vi "DLUInputBuffer.vi"(6 "Ready for Output":bool, 9 "Input Valid":bool, 10 "Input Data":T1) -> (1 "Output Data":bool, 2 "Output Data":T1, 4 "Ready For Input":bool)   [LabVIEW 2014, in "IO Node Logic Template.lvlib"]
uses:
  IO Node Logic Template.lvlib
  Node/Controls/Node_Command_Sent.ctl
  <vilib>/rvi/Emulation/niFpgaSctlEmulationGetInTimedLoop.vi
  <vilib>/rvi/DataTransferAndStorage/Container/Common/niFpgaContainerGetUniqueNameForEmu.vi
  <vilib>/rvi/DataTransferAndStorage/Container/Common/niFpgaContainerSetEmuInfo.vi
  <vilib>/rvi/eio/common/nirviEmuReportErrorAndStop.vi
  <vilib>/rvi/DataTransferAndStorage/Container/Common/niFpgaContainerExecOnDevCompGetState.vi
  <vilib>/rvi/Emulation/niFpgaEmulationIsFPGAContextNoSignature.vi
  <vilib>/rvi/errors/niFpgaSetErrorForExecOnDevCompSimple.vi
  <vilib>/rvi/FIFO/Fifo_Resource/nirvififoEmulationSetSize.vi
  <vilib>/rvi/FIFO/Fifo_Resource/nirviFifoEmulationQueueMgr.vi
  <instcachedir>/0/nirviFifoEmulationQueueMgr_E5CAEC123FF24DC58D834DCA3CDAA9B5.lvgen/nirviFifoEmulationQueueMgr_E5CAEC123FF24DC58D834DCA3CDAA9B5_001.vi
  <vilib>/rvi/FIFO/Fifo_Resource/nirvififoEmulationDetermineInputValidOut.vi
  <vilib>/rvi/FIFO/Fifo_Resource/nirvififoEmulationCreateLock.vi
  <vilib>/rvi/Emulation/niFpgaProcessEmulError.vi
  <vilib>/rvi/FIFO/Fifo_Resource/nirvififoEmulationObtainLock.vi
  <vilib>/rvi/FIFO/Fifo_Resource/nirvififoEmulationReleaseLock.vi
  <vilib>/rvi/occurrence/nirviWaitOnOccurrenceBase.vi
  <vilib>/rvi/errors/nirviReportUnexpectedCaseInternalError.vi
  <vilib>/rvi/errors/nirviReportUnexpectedCaseInternalError (U32).vi
  <vilib>/rvi/interface/RandomDataEmulation/niFpgaRandomDataHandleErrors.vi
  <vilib>/rvi/LocalResourceManager/LocalResourceManager.xnode
  <vilib>/rvi/DataTransferAndStorage/Container/XNode/niFpgaContainer.xnode
  <vilib>/rvi/FIFO/Fifo_Resource/niFpgaFifoEmulationRefIn.vi
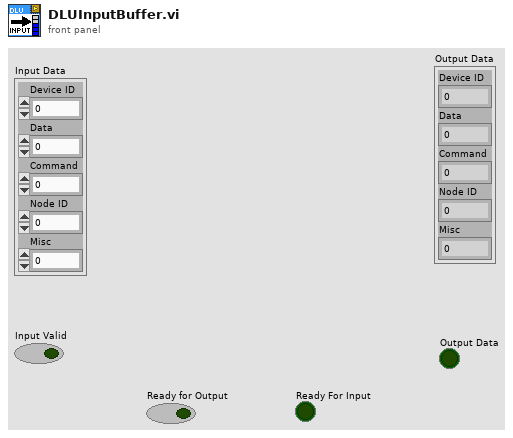
[diagram p1: front panel]
types:
  T1 = typedef "IO Node Logic Template.lvlib/Node_Command_Sent.ctl" = cluster{"Device ID":u8, "Data":u64, "Command":u8, "Node ID":u8, "Misc":u8}
  T2 = cluster{"Channel ID":u8, "Data":u64, "Command":u8, "Sender Address":u8, "Misc":u8}
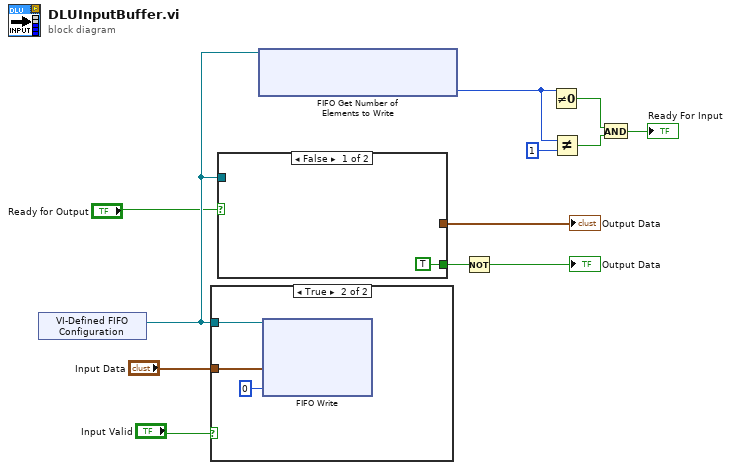
[diagram p0: block diagram]
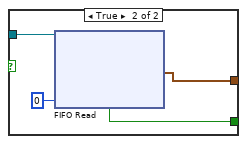
[diagram p2: hidden frame]
diagram:
  n1 = xnode "VI-Defined FIFO Configuration"() -> ("FIFO Out"=w8:refnum<k21>)
  n2 = case shown="True" "Input Valid" {
    tunnel: "Input Data" -> [_ w15]
    tunnel: w8 -> [_ w13]
    frame False {
    }
    frame True {
      n3 = xnode "FIFO Write"("Element"=w15, "Timeout"=0, "FIFO In"=w13) -> ()  [unwired: 2 out]
    }
  }
  n4 = case shown="False" "Ready for Output" {
    tunnel: [_ w19] -> w11
    tunnel: [TRUE ("Timed Out?") w18] -> w10
    tunnel: w8 -> [_ w17]
    frame False {
    }
    frame True {
      n5 = xnode "FIFO Read"("Timeout"=0, "FIFO In"=w17) -> ("Element"=w19:T2, "Timed Out?"=w18:bool)  [unwired: 1 out]
    }
  }
  "Output Data" <- w11
  n6 = xnode "FIFO Get Number of Elements to Write"("FIFO In"=w8) -> ("Number of Elements to Write"=w7:u32)  [unwired: 1 out]
  n7 = Not(x=w10) -> (.not. x?=→"Output Data":bool)
  n8 = Not Equal To 0?(x=w7) -> (x != 0?=w5:bool)
  n9 = Not Equal?(x=w7, y=u32 1) -> (x != y?=w6:bool)
  n10 = And(x=w5, y=w6) -> (x .and. y?=→"Ready For Input":bool)
